vi "DataProcess1.vi"(0 "DIO Group 1":T1={"Channel 1"=0, "Enable"=TRUE, "Main Switch"=0, "Channel 2"=0, "Channel 9"=0, "Channel 10"=0, "Channel 11"=0, "Channel 3"=0, "Channel 4"=0, "Channel 12"=0, "Channel 5"=0, "Channel 13"=0, "Channel 6"=0, "Channel 14"=0, "Channel 7"=0, "Channel 15"=0, "Channel 8"=0, "Channel 16"=0} caption="Data In") -> (1 "High Out":u16, 2 "Low Out":u16)   [LabVIEW 2012]
uses:
  ChannelStateControl.ctl
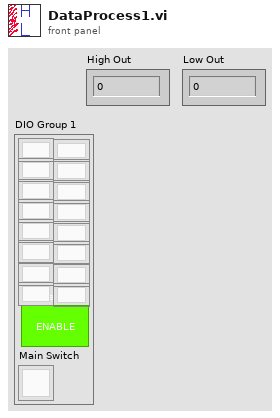
[diagram p1: front panel]
types:
  T1 = typedef "ChannelStateControl.ctl" = cluster{"Channel 1":u8, "Enable":bool, "Main Switch":u8, "Channel 2":u8, "Channel 9":u8, "Channel 10":u8, "Channel 11":u8, "Channel 3":u8, "Channel 4":u8, "Channel 12":u8, "Channel 5":u8, "Channel 13":u8, "Channel 6":u8, "Channel 14":u8, "Channel 7":u8, "Channel 15":u8, "Channel 8":u8, "Channel 16":u8}
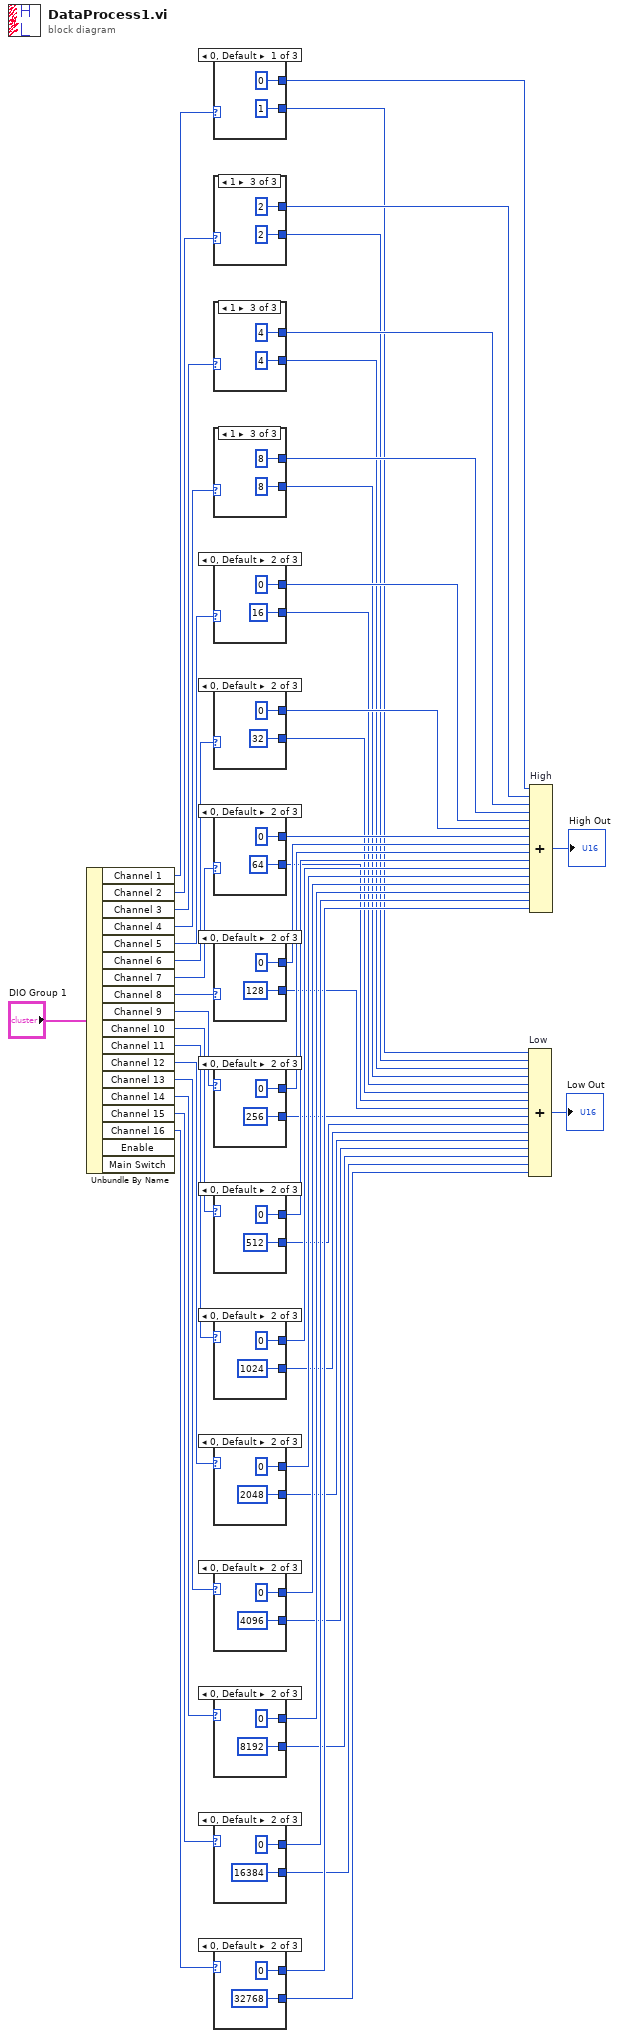
[diagram p0: block diagram]
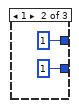
[diagram p2: hidden frame]
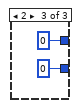
[diagram p3: hidden frame]
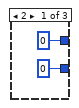
[diagram p4: hidden frame]
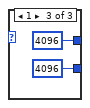
[diagram p5: hidden frame]
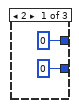
[diagram p6: hidden frame]
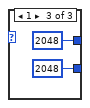
[diagram p7: hidden frame]
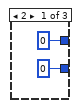
[diagram p8: hidden frame]
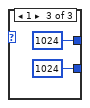
[diagram p9: hidden frame]
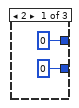
[diagram p10: hidden frame]
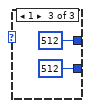
[diagram p11: hidden frame]
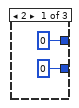
[diagram p12: hidden frame]
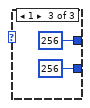
[diagram p13: hidden frame]
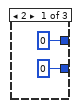
[diagram p14: hidden frame]
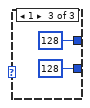
[diagram p15: hidden frame]
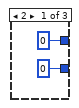
[diagram p16: hidden frame]
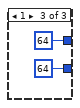
[diagram p17: hidden frame]
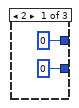
[diagram p18: hidden frame]
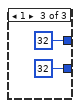
[diagram p19: hidden frame]
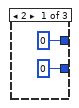
[diagram p20: hidden frame]
diagram:
  n1 = Unbundle By Name("DIO Group 1") -> ("Channel 1"=w51:u8, "Channel 2"=w50:u8, "Channel 3"=w49:u8, "Channel 4"=w48:u8, "Channel 5"=w47:u8, "Channel 6"=w46:u8, "Channel 7"=w45:u8, "Channel 8"=w44:u8, "Channel 9"=w43:u8, "Channel 10"=w42:u8, "Channel 11"=w41:u8, "Channel 12"=w40:u8, "Channel 13"=w39:u8, "Channel 14"=w38:u8, "Channel 15"=w37:u8, "Channel 16"=w36:u8)  [unwired: 2 out]
  n2 = case shown="0, Default" w51 {
    tunnel: [u16 0 u16 1 u16 0] -> w35
    tunnel: [u16 1 u16 1 u16 0] -> w19
    frame 0, Default {
    }
    frame 1 {
    }
    frame 2 {
    }
  }
  n3 = case shown="1" w50 {
    tunnel: [u16 0 u16 0 u16 2] -> w34
    tunnel: [u16 0 u16 2 u16 2] -> w18
    frame 2 {
    }
    frame 0, Default {
    }
    frame 1 {
    }
  }
  n4 = case shown="1" w49 {
    tunnel: [u16 0 u16 0 u16 4] -> w33
    tunnel: [u16 0 u16 4 u16 4] -> w17
    frame 2 {
    }
    frame 0, Default {
    }
    frame 1 {
    }
  }
  n5 = case shown="1" w48 {
    tunnel: [u16 0 u16 0 u16 8] -> w32
    tunnel: [u16 0 u16 8 u16 8] -> w16
    frame 2 {
    }
    frame 0, Default {
    }
    frame 1 {
    }
  }
  n6 = case shown="0, Default" w47 {
    tunnel: [u16 0 u16 0 u16 16] -> w31
    tunnel: [u16 0 u16 16 u16 16] -> w15
    frame 2 {
    }
    frame 0, Default {
    }
    frame 1 {
    }
  }
  n7 = case shown="0, Default" w46 {
    tunnel: [u16 0 u16 0 u16 32] -> w30
    tunnel: [u16 0 u16 32 u16 32] -> w14
    frame 2 {
    }
    frame 0, Default {
    }
    frame 1 {
    }
  }
  n8 = case shown="0, Default" w45 {
    tunnel: [u16 0 u16 0 u16 64] -> w29
    tunnel: [u16 0 u16 64 u16 64] -> w13
    frame 2 {
    }
    frame 0, Default {
    }
    frame 1 {
    }
  }
  n9 = case shown="0, Default" w44 {
    tunnel: [u16 0 u16 0 u16 128] -> w28
    tunnel: [u16 0 u16 128 u16 128] -> w12
    frame 2 {
    }
    frame 0, Default {
    }
    frame 1 {
    }
  }
  n10 = case shown="0, Default" w43 {
    tunnel: [u16 0 u16 0 u16 256] -> w27
    tunnel: [u16 0 u16 256 u16 256] -> w11
    frame 2 {
    }
    frame 0, Default {
    }
    frame 1 {
    }
  }
  n11 = case shown="0, Default" w42 {
    tunnel: [u16 0 u16 0 u16 512] -> w26
    tunnel: [u16 0 u16 512 u16 512] -> w10
    frame 2 {
    }
    frame 0, Default {
    }
    frame 1 {
    }
  }
  n12 = case shown="0, Default" w41 {
    tunnel: [u16 0 u16 0 u16 1024] -> w25
    tunnel: [u16 0 u16 1024 u16 1024] -> w9
    frame 2 {
    }
    frame 0, Default {
    }
    frame 1 {
    }
  }
  n13 = case shown="0, Default" w40 {
    tunnel: [u16 0 u16 0 u16 2048] -> w24
    tunnel: [u16 0 u16 2048 u16 2048] -> w8
    frame 2 {
    }
    frame 0, Default {
    }
    frame 1 {
    }
  }
  n14 = case shown="0, Default" w39 {
    tunnel: [u16 0 u16 0 u16 4096] -> w23
    tunnel: [u16 0 u16 4096 u16 4096] -> w7
    frame 2 {
    }
    frame 0, Default {
    }
    frame 1 {
    }
  }
  n15 = case shown="0, Default" w38 {
    tunnel: [u16 0 u16 0 u16 8192] -> w22
    tunnel: [u16 0 u16 8192 u16 8192] -> w6
    frame 2 {
    }
    frame 0, Default {
    }
    frame 1 {
    }
  }
  n16 = case shown="0, Default" w37 {
    tunnel: [u16 0 u16 0 u16 16384] -> w21
    tunnel: [u16 0 u16 16384 u16 16384] -> w5
    frame 2 {
    }
    frame 0, Default {
    }
    frame 1 {
    }
  }
  n17 = case shown="0, Default" w36 {
    tunnel: [u16 0 u16 0 u16 32768] -> w20
    tunnel: [u16 0 u16 32768 u16 32768] -> w4
    frame 2 {
    }
    frame 0, Default {
    }
    frame 1 {
    }
  }
  n18 = Compound Arithmetic op=ADD "Low"(w19, w18, w17, w16, w15, w14, w13, w12, w11, w10, w9, w8, w7, w6, w5, w4) -> (→"Low Out":u16)
  n19 = Compound Arithmetic op=ADD "High"(w35, w34, w33, w32, w31, w30, w29, w28, w27, w26, w25, w24, w23, w22, w21, w20) -> (→"High Out":u16)
